vi "ui get duplicate jpg file name list.vi"() -> ()   [LabVIEW 2023]
panel:
  out "FIltered file count":i32
  out "Total file count":i32
  in  "Root folder path of all files":path
  out "Destination":path[](array[path])
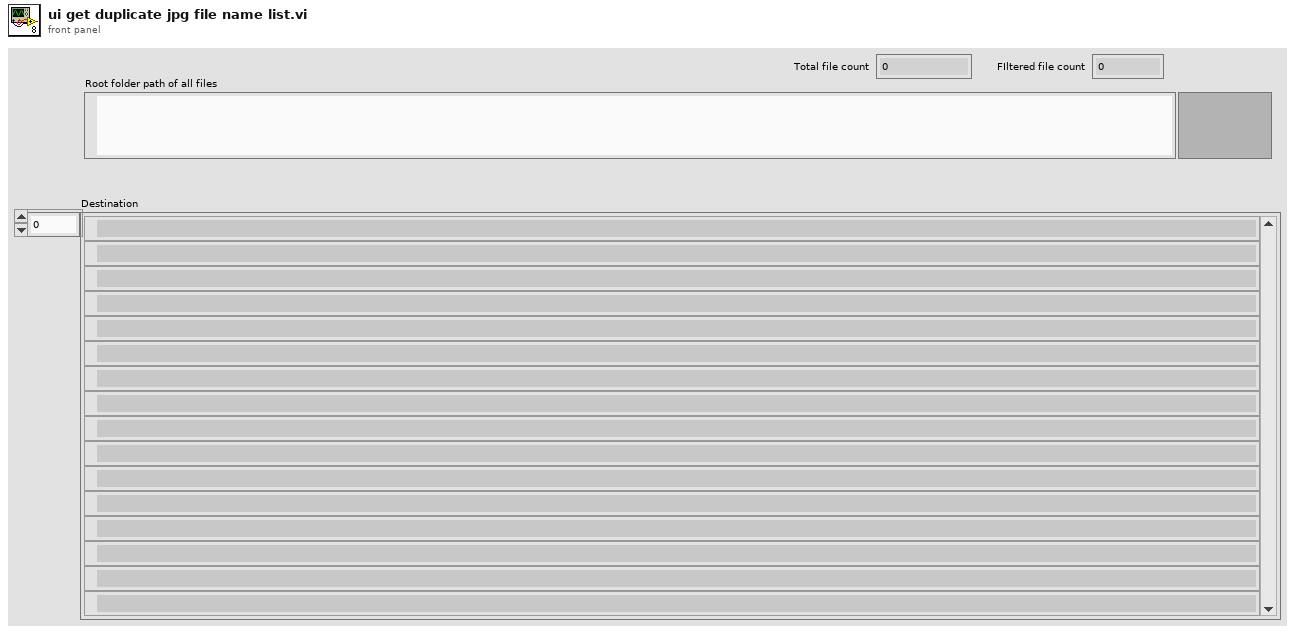
[diagram p1: front panel]
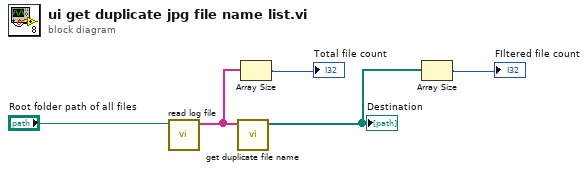
[diagram p0: block diagram]
diagram:
  n1 = call "read log file.vi"("file (use dialog)"="Root folder path of all files") -> ("array"=w4:string[])  [unwired: 10 in]
  n2 = call "get duplicate file name.vi"("path list"=w4) -> ("Array"=w1:path[])  [unwired: 10 in]
  "Destination" <- w1
  n3 = Array Size(array=w4) -> (size(s)=→"Total file count":i32)
  n4 = Array Size(array=w1) -> (size(s)=→"FIltered file count":i32)
